vi "practica112.vi"() -> ()   [LabVIEW 2013]
uses:
  <vilib>/Native 3D Graph/xcontrol/3DPC_SurfacePlot.xctl
panel:
  in  "eje z":dbl
  out "3D Graph":refnum<class "Base Datatype.lvclass">[](xcontrol)
  out "S2 x":dbl
  out "S2 y":dbl
  out "S1 x":dbl
  out "S1 y":dbl
  in  "S2":i32
  in  "S1":i32
  in  "stop":bool
  in  "S2":dbl(knob) scale=-175.0..175.0
  in  "S1":dbl(knob) scale=0.0..360.0
  out "XY Graph":cluster{"Y":dbl[], "Y":dbl[]}[](graph)
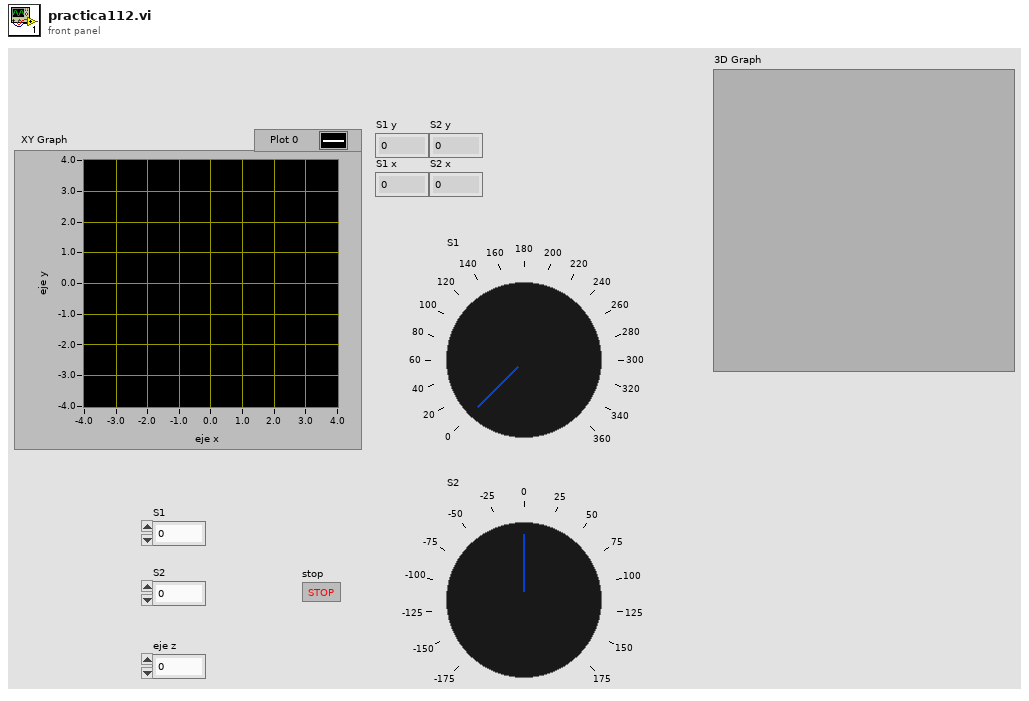
[diagram p1: front panel]
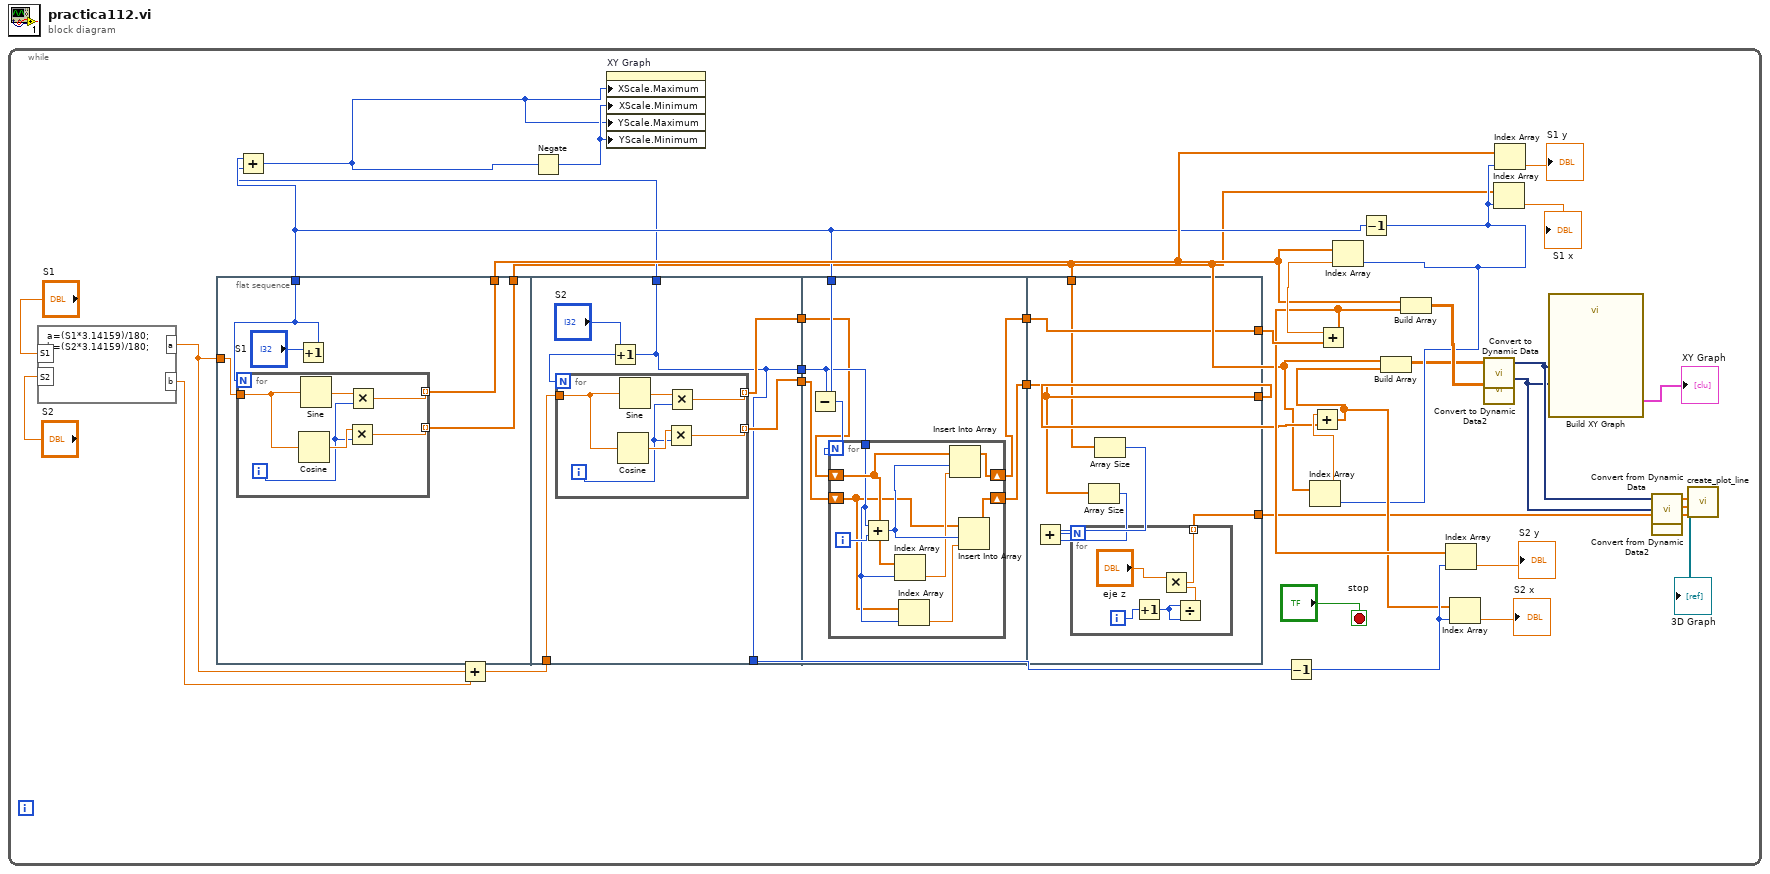
[diagram p0: block diagram]
diagram:
  n1 = while {
    stop <- "stop" stop-if-true
    n2 = formula code="a=(S1*3.14159)/180;\nb=(S2*3.14159)/180;"("S1"="S1", "S2"="S2") -> ("b"=w33:dbl, "a"=w32:dbl)
    n3 = flat-sequence {
      tunnel: w32 -> [w44]
      tunnel: [w40] -> w16
      tunnel: [w42] -> w26
      tunnel: [w41] -> w7
      tunnel: w31 -> [w54]
      tunnel: [w53] -> w29
      tunnel: [w52] -> w28
      tunnel: [w51] -> w27
      tunnel: [w51] -> w19
      tunnel: [w51] -> w15
      tunnel: w29 -> [w62]
      tunnel: w28 -> [w63]
      tunnel: w16 -> [w68]
      tunnel: w27 -> [w66]
      tunnel: [w64] -> w10
      tunnel: [w65] -> w9
      tunnel: [w81] -> w23
      tunnel: [w80] -> w8
      tunnel: w10 -> [w80]
      tunnel: w9 -> [w81]
      tunnel: w7 -> [w79]
      tunnel: [w78] -> w6
      frame #0 {
        n4 = Increment(x="S1") -> (x+1=w40:i32)
        n5 = for {
          N: w40 -> [_]
          tunnel: w44 -> [w46]
          tunnel: [w48] -> w42 mode=indexing
          tunnel: [w47] -> w41 mode=indexing
          i -> [w45]
          n6 = Cosine(x=w46) -> (cos(x)=w50:dbl)
          n7 = Sine(x=w46) -> (sin(x)=w49:dbl)
          n8 = Multiply(x=w50, y=w45) -> (x*y=w47:dbl)
          n9 = Multiply(x=w49, y=w45) -> (x*y=w48:dbl)
        }
      }
      frame #1 {
        n10 = Increment(x="S2") -> (x+1=w51:i32)
        n11 = for {
          N: w51 -> [_]
          tunnel: w54 -> [w57]
          tunnel: [w59] -> w52 mode=indexing
          tunnel: [w58] -> w53 mode=indexing
          i -> [w56]
          n12 = Cosine(x=w57) -> (cos(x)=w61:dbl)
          n13 = Sine(x=w57) -> (sin(x)=w60:dbl)
          n14 = Multiply(x=w61, y=w56) -> (x*y=w58:dbl)
          n15 = Multiply(x=w60, y=w56) -> (x*y=w59:dbl)
        }
      }
      frame #2 {
        n16 = Subtract(x=w68, y=w66) -> (x-y=w67:i32)
        n17 = for {
          N: w67 -> [_]
          tunnel: w66 -> [w72]
          shift-right: [w73] -> w65
          shift-left: w63 -> [w75]
          shift-right: [w69] -> w64
          shift-left: w62 -> [w71]
          i -> [w77]
          n18 = Add(x=w72, y=w77) -> (x+y=w76:i32)
          n19 = Index Array(array=w75, index=w72) -> (element=w74:dbl)
          n20 = Index Array(array=w71, index=w72) -> (element=w70:dbl)
          n21 = Insert Into Array(array=w75, index=w76, new element=w74) -> (w73:dbl[])
          n22 = Insert Into Array(array=w71, index=w76, new element=w70) -> (w69:dbl[])
        }
      }
      frame #3 {
        n23 = Array Size(array=w80) -> (size(s)=w83:i32)
        n24 = Array Size(array=w79) -> (size(s)=w84:i32)
        n25 = Add(x=w84, y=w83) -> (x+y=w82:i32)
        n26 = for {
          N: w82 -> [_]
          tunnel: [w87] -> w78 mode=indexing
          i -> [w86]
          n27 = Increment(x=w86) -> (x+1=w85:i32)
          n28 = Divide(x=w85, y=w85) -> (x/y=w89:dbl)
          n29 = Multiply(x="eje z", y=w89) -> (x*y=w87:dbl)
        }
      }
    }
    n30 = Add(x=w16, y=w15) -> (x+y=w13:i32)
    n31 = Add(x=w32, y=w33) -> (x+y=w31:dbl)
    n32 = Negate(x=w13) -> (-x=w14:i32)
    n33 = property on="XY Graph" class="XYGraph (strict)"("XScale.Maximum"=w13, "XScale.Minimum"=w14, "YScale.Maximum"=w13, "YScale.Minimum"=w14) -> ()  [unwired: 2 in, 2 out]
    n34 = Decrement(x=w19) -> (x-1=w20:i32)
    n35 = Decrement(x=w16) -> (x-1=w11:i32)
    n36 = Index Array(array=w7, index=w11) -> (element=w34:dbl)
    n37 = Add(x=w34, y=w8) -> (x+y=w17:dbl[])
    n38 = Index Array(array=w26, index=w11) -> (element=w30:dbl)
    n39 = Add(x=w30, y=w23) -> (x+y=w18:dbl[])
    n40 = Build Array(w7, w17) -> (w5:dbl[][])
    n41 = Build Array(w26, w18) -> (w36:dbl[][])
    n42 = Index Array(array=w18, index=w20) -> (element=→"S2 y":dbl)
    n43 = Index Array(array=w17, index=w20) -> (element=→"S2 x":dbl)
    n44 = call "Convert to Dynamic Data"("2D Array"=w5) -> ("Dynamic Data Type"=w4:dynamicdata)  [unwired: 3 in]
    n45 = call "Convert to Dynamic Data2"("2D Array"=w36) -> ("Dynamic Data Type"=w2:dynamicdata)  [unwired: 3 in]
    n46 = Index Array(array=w7, index=w11) -> (element=→"S1 x":dbl)
    n47 = Index Array(array=w26, index=w11) -> (element=→"S1 y":dbl)
    n48 = call "Build XY Graph"("Y Input"=w2, "X Input"=w4) -> ("XY Graph"=→"XY Graph":cluster{"X":dbl[], "Y":dbl[]}[])  [unwired: 8 in, 1 out]
    n49 = call "Convert from Dynamic Data"("Dynamic Data Type"=w4) -> ("Array"=w3:dbl[])  [unwired: 3 in]
    n50 = call "Convert from Dynamic Data2"("Dynamic Data Type"=w2) -> ("Array"=w1:dbl[])  [unwired: 3 in]
    n51 = call <vilib>:"create_plot_line.vi"("z vector"=w6, "y vector"=w1, "x vector"=w3) -> ("plots out"=→"3D Graph":refnum<class "Base Datatype.lvclass">[])  [unwired: 2 in, 6 out]
  }
